vi "Update System Log String.vi"(8 "error in (no error)":errorcluster, 10 "Message In":string, 11 "UI 1 Data in":T1={"System Log"="", "[Array Of Threshold Refs]"=[], "[Array Of Boarder Refs]"=[], "APU Type"="", "APU Setup File"={"Sensor Info"=[], "Variables"=[], "CMM Table 106"=[], "CMM Table 106B "=[], "Accel Config"=[], "Report Sheet 1"=[], "Report Sheet 2"=[], "Report Sheet 3"=[]}, "ActiveValuetoRecordRow"=[], "ReportType"=[], "ReportValue"=[], "ActiveReportSheets"=[], "APUOn"=FALSE, "APUOnTime"=timestamp(0 s since 1904-01-01), "APUOffTime"=timestamp(0 s since 1904-01-01), "Recording"=FALSE, "Test Information"={"APU Part Number:"="555", "Model:"="5", "Serial Number:"="sad", "Customer:"="sad", "Work Order:"="asd", "Pre or Post SB"="Pre SB 49-7711", "Run Count"=0, "APU Selected"="<Select>"}, "APU RUN TIME"=timestamp(0 s since 1904-01-01)} {"APU RUN TIME" format="%<%H:%M:%S>T"; "Test Information"."Run Count" min=0 step=1; "APUOffTime" format="%<%x %.3X>T"; "APUOnTime" format="%<%x %.3X>T"}) -> (0 "error out":errorcluster, 2 "System Log":string, 3 "UI 1 Data out":T1={"System Log"="", "[Array Of Threshold Refs]"=[], "[Array Of Boarder Refs]"=[], "APU Type"="", "APU Setup File"={"Sensor Info"=[], "Variables"=[], "CMM Table 106"=[], "CMM Table 106B "=[], "Accel Config"=[], "Report Sheet 1"=[], "Report Sheet 2"=[], "Report Sheet 3"=[]}, "ActiveValuetoRecordRow"=[], "ReportType"=[], "ReportValue"=[], "ActiveReportSheets"=[], "APUOn"=FALSE, "APUOnTime"=timestamp(0 s since 1904-01-01), "APUOffTime"=timestamp(0 s since 1904-01-01), "Recording"=FALSE, "Test Information"={"APU Part Number:"="555", "Model:"="5", "Serial Number:"="sad", "Customer:"="sad", "Work Order:"="asd", "Pre or Post SB"="Pre SB 49-7711", "Run Count"=0, "APU Selected"="<Select>"}, "APU RUN TIME"=timestamp(0 s since 1904-01-01)} {"APU RUN TIME" format="%<%H:%M:%S>T"; "Test Information"."Run Count" min=0 step=1; "APUOffTime" format="%<%x %.3X>T"; "APUOnTime" format="%<%x %.3X>T"})   [LabVIEW 2018, in "Testing UI 1.lvlib"]
uses:
  Testing UI 1.lvlib
  Private Controls/UI 1 Data.ctl
  Top Level/Shared Controls/APU Setup File.ctl
  File IO/Public Controls/ReportType.ctl
  Controller (Host)/Public Controls/Test Information.ctl
  Controller (Host)/Public VIs/PreorPostSB.ctl
  Controller (Host)/Public Controls/APU Select.ctl
  File IO/File IO.lvlib
  Controller (Host)/Controller (Host).lvlib
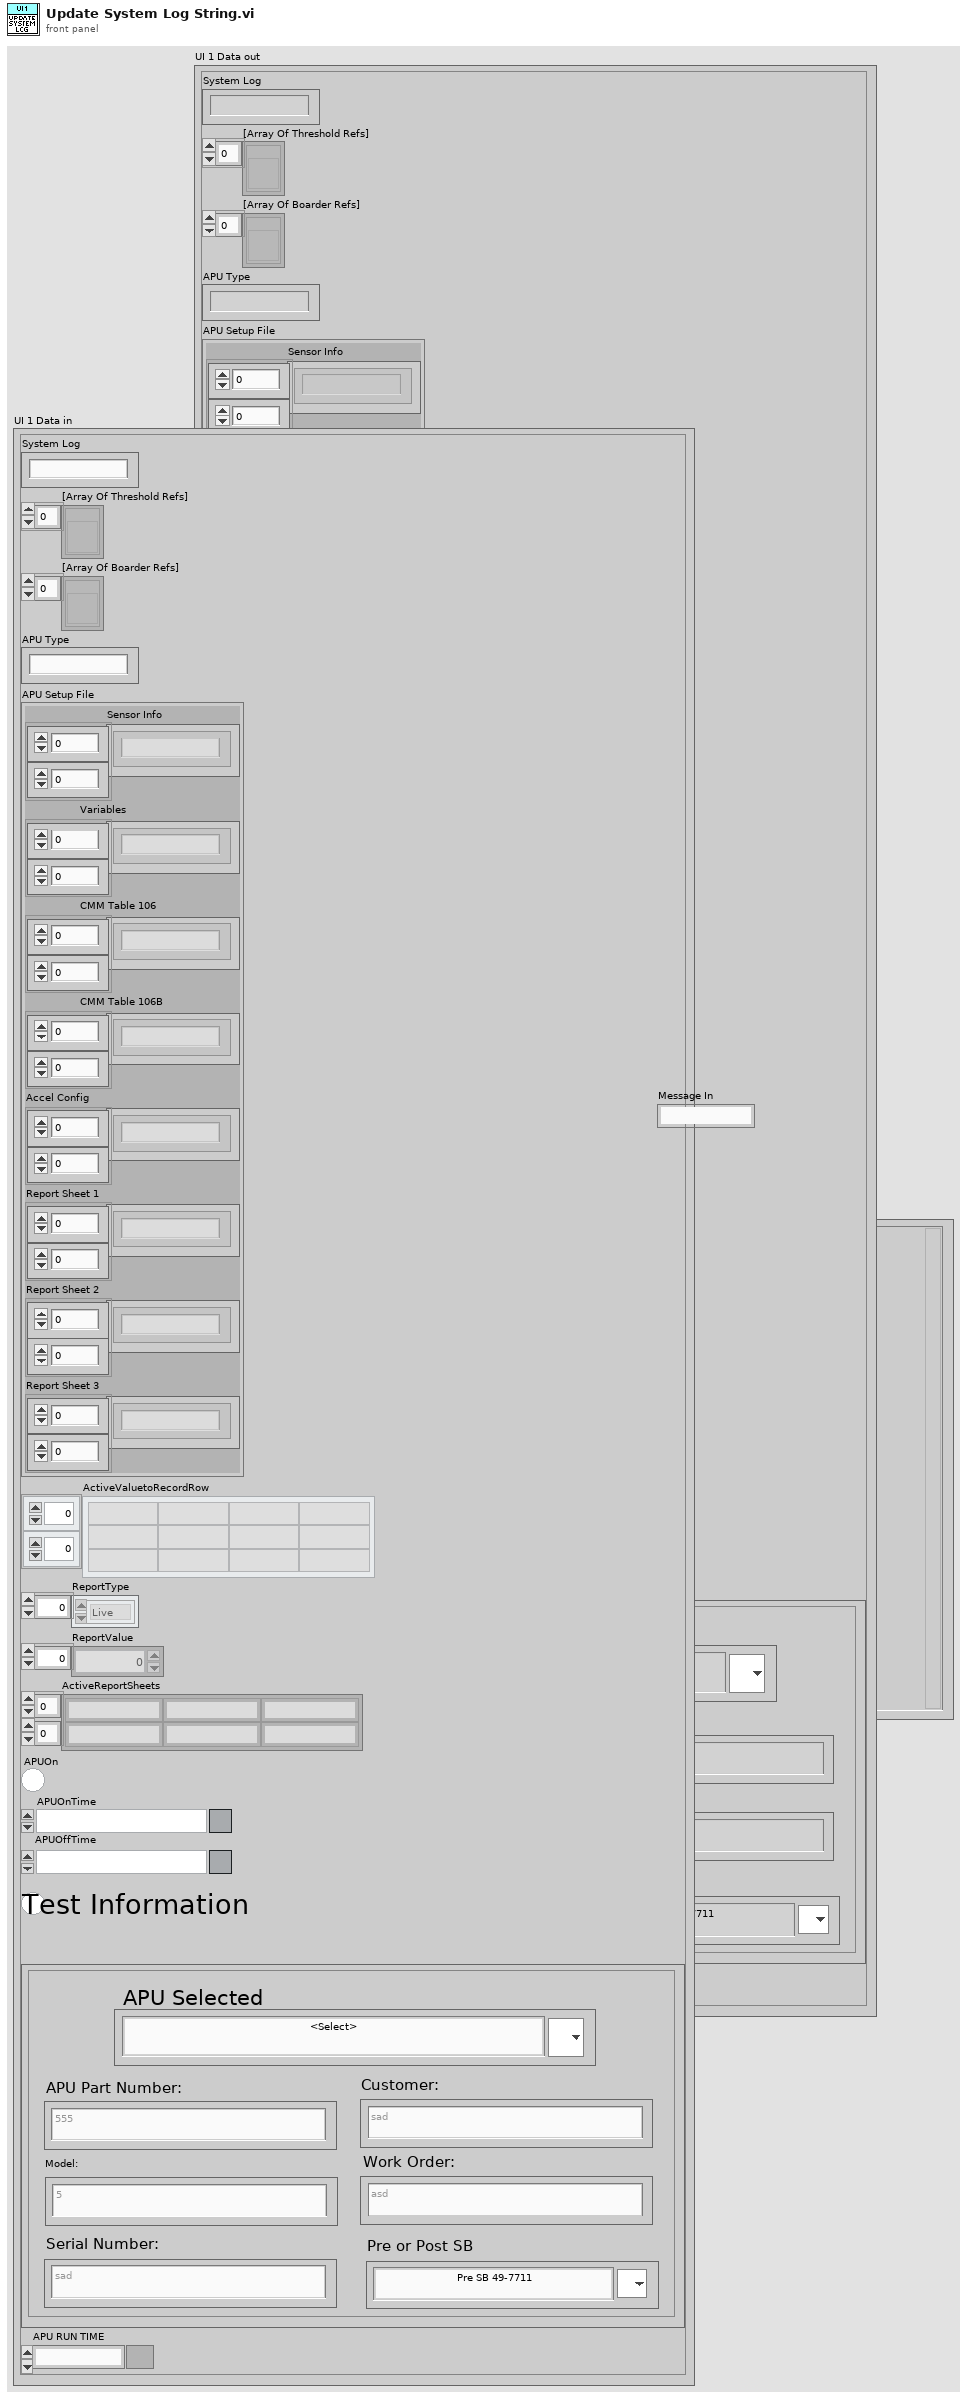
[diagram p1: front panel]
types:
  T1 = typedef "Testing UI 1.lvlib/UI 1 Data.ctl" = cluster{"System Log":string, "[Array Of Threshold Refs]":refnum<vi>[], "[Array Of Boarder Refs]":refnum<vi>[], "APU Type":string, "APU Setup File":T2, "ActiveValuetoRecordRow":string[][], "ReportType":T3[], "ReportValue":dbl[], "ActiveReportSheets":string[][], "APUOn":bool, "APUOnTime":timestamp, "APUOffTime":timestamp, "Recording":bool, "Test Information":T4, "APU RUN TIME":timestamp}
  T2 = typedef "APU Setup File.ctl" = cluster{"Sensor Info":string[][], "Variables":string[][], "CMM Table 106":string[][], "CMM Table 106B ":string[][], "Accel Config":string[][], "Report Sheet 1":string[][], "Report Sheet 2":string[][], "Report Sheet 3":string[][]}
  T3 = typedef "File IO.lvlib/ReportType.ctl" = enum16{"Live", "Min", "Max", "Deviation"}
  T4 = typedef "Controller (Host).lvlib/Test Information.ctl" = cluster{"APU Part Number:":string, "Model:":string, "Serial Number:":string, "Customer:":string, "Work Order:":string, "Pre or Post SB":T5, "Run Count":i32, "APU Selected":T6}
  T5 = typedef "Controller (Host).lvlib/PreorPostSB.ctl" = string
  T6 = typedef "Controller (Host).lvlib/APU Select.ctl" = string
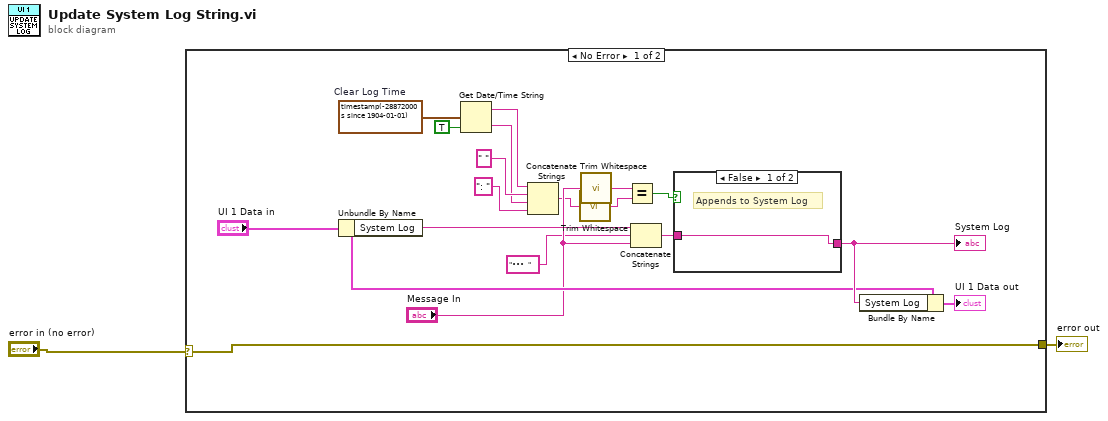
[diagram p0: block diagram]
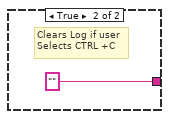
[diagram p2: hidden frame]
diagram:
  n1 = case shown="No Error" "error in (no error)" {
    selector: "error in (no error)" -> [w8 w23]
    tunnel: [w8 w23] -> w1
    frame No Error {
      w9 = timestamp(-28872000 s since 1904-01-01)  # Clear Log Time
      n2 = Unbundle By Name("UI 1 Data in") -> ("System Log"=w15:string)
      n3 = Get Date/Time String(seconds (now)=w9, want seconds? (F)=TRUE) -> (date string=w11:string, time string=w13:string)  [unwired: 1 in]
      n4 = Concatenate Strings(w11, " " ("string"), w13, ": " ("string")) -> (w4:string)
      n5 = call <vilib>:"Trim Whitespace.vi"("string"=w4) -> ("trimmed string"=w3:string)  [unwired: 1 in]
      n6 = call <vilib>:"Trim Whitespace.vi"("string"="Message In") -> ("trimmed string"=w5:string)  [unwired: 1 in]
      n7 = Equal?(x=w5, y=w3) -> (x = y?=w20:bool)
      n8 = Concatenate Strings(w15, "•••  " ("string"), "Message In") -> (w19:string)
      n9 = case shown="False" w20 {
        tunnel: [w21 ""] -> w18
        tunnel: w19 -> [w21 _]
        frame False {
          # "Appends to System Log"
        }
        frame True {
          # "Clears Log if user\nSelects CTRL +C"
        }
      }
      "System Log" <- w18
      n10 = Bundle By Name(cluster="UI 1 Data in", "System Log"=w18) -> (→"UI 1 Data out":T1)
    }
    frame Error {
      # "Propogate error through subvi"
    }
  }
  "error out" <- w1
